vi "Lean Angle Adjustment.vi"(9 "Velocity":dbl, 11 "Value Channel 0":i32) -> (2 "Reference lean angle":dbl)   [LabVIEW 2016]
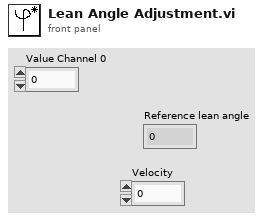
[diagram p1: front panel]
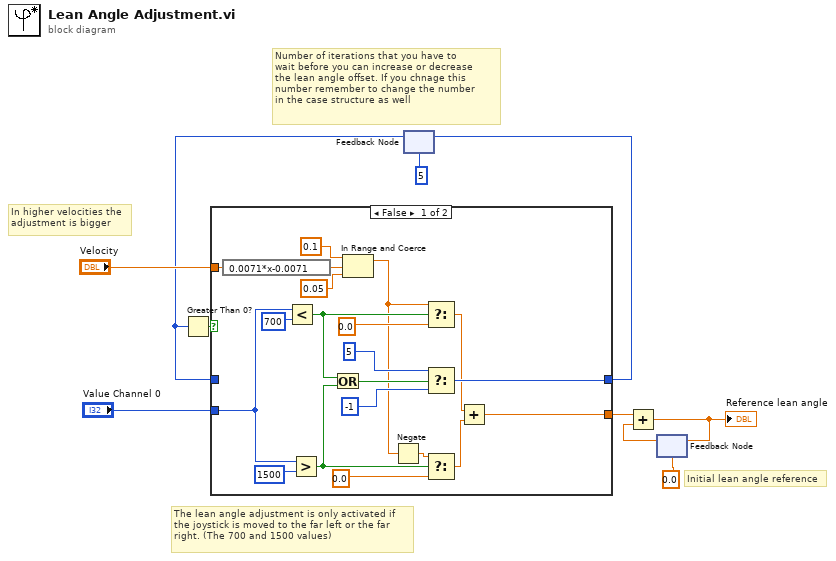
[diagram p0: block diagram]
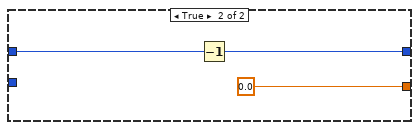
[diagram p2: hidden frame]
diagram:
  # "The lean angle adjustment is only activated if\nthe joystick is moved to the far left or the far\nright. (The 700 and 1500 values)"
  # "In higher velocities the\nadjustment is bigger"
  # "Number of iterations that you have to\nwait before you can increase or decrease\nthe lean angle offset. If you chnage this \nnumber remember to change the number \nin the case structure as well"
  # "Initial lean angle reference"
  n1 = feedback #1(5 ("f")) -> (w2:i32)
  n2 = Greater Than 0?(x=w2) -> (x > 0?=w9:bool)
  n3 = case shown="False" w9 {
    tunnel: w2 -> [_ w33]
    tunnel: [w25 w32] -> w3
    tunnel: "Value Channel 0" -> [w28 _]
    tunnel: [w17 0.0] -> w10
    tunnel: "Velocity" -> [w11 _]
    frame False {
      n4 = expression code="0.0071*x-0.0071"(w11) -> (w14:dbl)
      n5 = Less?(x=w28, y=700 ("upper limit")) -> (x < y?=w23:bool)
      n6 = Greater?(x=w28, y=1500 ("upper limit")) -> (0:w21:bool)
      n7 = Or(x=w23, y=w21) -> (x .or. y?=w27:bool)
      n8 = In Range and Coerce(upper limit=0.1, x=w14, lower limit=0.05) -> (coerced(x)=w12:dbl)  [unwired: 1 out]
      n9 = Negate(x=w12) -> (-x=w13:dbl)
      n10 = Select(t=w12, s=w23, f=0.0) -> (s? t:f=w19:dbl)
      n11 = Select(t=5, s=w27, f=-1) -> (s? t:f=w25:i32)
      n12 = Select(t=w13, s=w21, f=0.0) -> (s? t:f=w18:dbl)
      n13 = Add(x=w19, y=w18) -> (x+y=w17:dbl)
    }
    frame True {
      n14 = Decrement(x=w33) -> (x-1=w32:i32)
    }
  }
  n15 = feedback-in #1(w3) -> ()
  n16 = feedback #2(0.0) -> (w5:dbl)
  n17 = Add(x=w10, y=w5) -> (x+y=w6:dbl)
  "Reference lean angle" <- w6
  n18 = feedback-in #2(w6) -> ()
